vi "CheckFileExist.vi"(7 "format string":string="%03d", 8 "error in (no error) 2":errorcluster, 10 "Interactive":bool=TRUE, 11 "File in":path) -> (0 "error out":errorcluster, 2 "Overwrite":bool, 3 "File out":path)   [LabVIEW 2021]
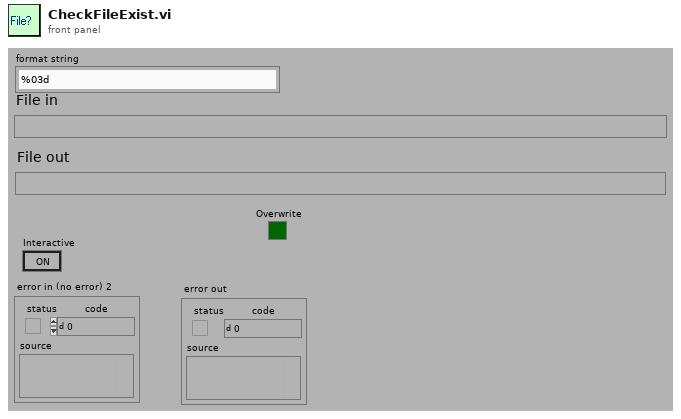
[diagram p1: front panel]
types:
  T1 = enum32{"existing file", "new file", "new or existing file", "existing dir", "new dir", "new or existing dir", "existing file (use LLBs)", "new file (use LLBs)", "new or existing file (use LLBs)", "new or existing file or directory (use LLBs)", "existing dir (use LLBs)", "new dir (use LLBs)", "new or existing dir (use LLBs)", "existing file or dir", "new file or dir", "new or existing file or dir", "existing file or dir (use LLBs)", "new file or dir (use LLBs)"}
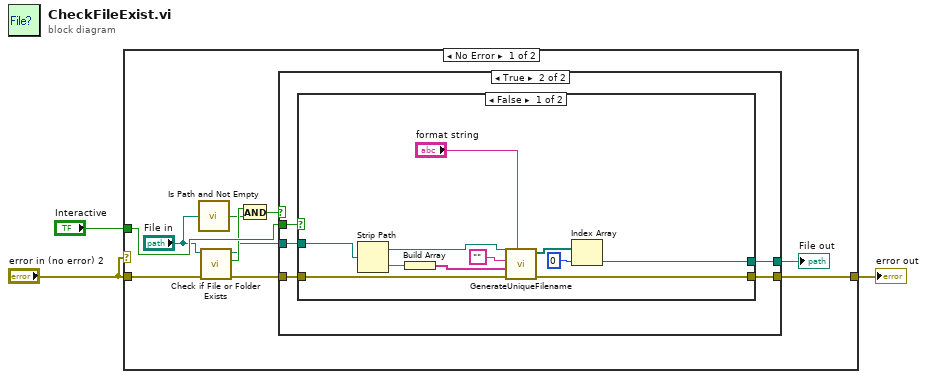
[diagram p0: block diagram]
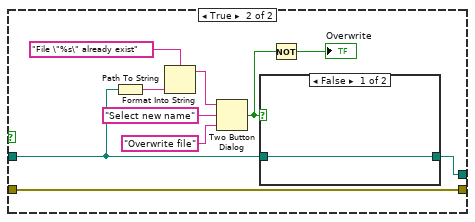
[diagram p3: hidden frame]
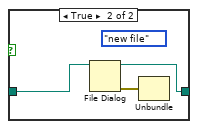
[diagram p4: hidden frame]
diagram:
  n1 = case shown="No Error" "error in (no error) 2" {
    tunnel: "Interactive" -> [w12 _]
    tunnel: [w11 w46] -> w2
    tunnel: "error in (no error) 2" -> [w9 w46]
    frame No Error {
      n2 = call <vilib>:"Is Path and Not Empty.vi"("path"="File in") -> ("Is Path and Not Empty?"=w6:bool)  [unwired: 4 in]
      n3 = call <vilib>:"Check if File or Folder Exists.vi"("error in (no error)"=w9, "path"="File in") -> ("error out"=w8:errorcluster, "file or folder exists?"=w10:bool, "dup path"=w4:path)  [unwired: 7 in]
      n4 = And(x=w10, y=w6) -> (x .and. y?=w7:bool)
      n5 = case shown="True" w7 {
        tunnel: w4 -> [w15 w19]
        tunnel: [w15 w20] -> w13
        tunnel: w12 -> [_ w18]
        tunnel: w8 -> [w14 w17]
        tunnel: [w14 w16] -> w11
        frame False {
        }
        frame True {
          n6 = case shown="False" w18 {
            tunnel: [w23 w41] -> w20
            tunnel: w19 -> [w31 w37]
            tunnel: w17 -> [w28 w33]
            tunnel: [w27 w33] -> w16
            frame False {
              n7 = Strip Path(path=w31) -> (stripped path=w30:path, name=w29:string)
              n8 = Build Array(w29) -> (w25:string[])
              n9 = call "GenerateUniqueFilename.vi"("format string"="format string", "Error In"=w28, "File name suffixes"=w25, "File name prefix"="", "Folder Path Control"=w30) -> ("Error Out"=w27:errorcluster, "Paths"=w26:path[])  [unwired: 2 in, 3 out]
              n10 = Index Array(array=w26, index=0) -> (element=w23:path)
            }
            frame True {
              n11 = Path To String(path=w37) -> (string=w36:string)
              n12 = Format Into String(format string="File \"%s\" already exist", w36) -> (resulting string=w34:string)  [unwired: 2 in, 1 out]
              n13 = Two Button Dialog(message=w34, 1:"Overwrite file", 2:"Select new name") -> (T button?=w38:bool)
              n14 = case shown="False" w38 {
                tunnel: [w42 w45] -> w41
                tunnel: w37 -> [w42 w44]
                frame False {
                }
                frame True {
                  (unwired) T1."new file" ("select mode (2)")
                  n15 = File Dialog(11:w44) -> (0:w43:errorcluster, 3:w45:path)  [unwired: 1 in, 7 out]
                  n16 = Unbundle(w43) -> ()  [unwired: 3 out]
                }
              }
              n17 = Not(x=w38) -> (.not. x?=→"Overwrite":bool)
            }
          }
        }
      }
      "File out" <- w13
    }
    frame Error {
    }
  }
  "error out" <- w2
